vi "PKDAQInsertBlockData.vi"(0 "Block Data":T1, 5 "C12":dbl, 7 "C13L":dbl, 9 "C13H":dbl, 11 "Counts":u32, 12 "LT":dbl, 13 "RT":dbl) -> (4 "Block Data Out":T1)   [LabVIEW 2011]
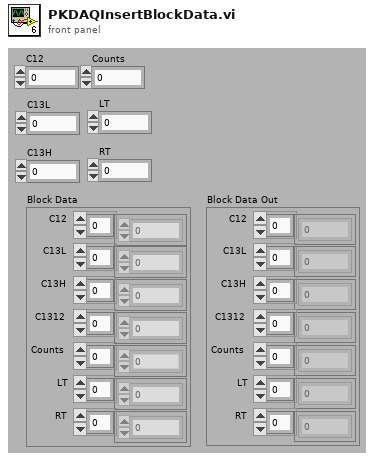
[diagram p1: front panel]
types:
  T1 = cluster{"C12":dbl[], "C13L":dbl[], "C13H":dbl[], "Counts":u32[], "LT":dbl[], "RT":dbl[], "C1312":dbl[]}
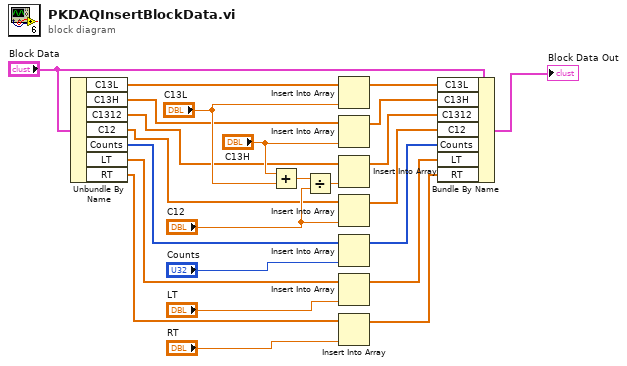
[diagram p0: block diagram]
diagram:
  n1 = Unbundle By Name("Block Data") -> ("C13L"=w4:dbl[], "C13H"=w1:dbl[], "C1312"=w3:dbl[], "C12"=w2:dbl[], "Counts"=w20:u32[], "LT"=w19:dbl[], "RT"=w18:dbl[])
  n2 = Add(x="C13H", y="C13L") -> (x+y=w10:dbl)
  n3 = Divide(x=w10, y="C12") -> (x/y=w9:dbl)
  n4 = Insert Into Array(array=w4, new element="C13L") -> (w5:dbl[])  [unwired: 1 in]
  n5 = Insert Into Array(array=w1, new element="C13H") -> (w6:dbl[])  [unwired: 1 in]
  n6 = Insert Into Array(array=w3, new element=w9) -> (w7:dbl[])  [unwired: 1 in]
  n7 = Insert Into Array(array=w2, new element="C12") -> (w8:dbl[])  [unwired: 1 in]
  n8 = Insert Into Array(array=w20, new element="Counts") -> (w17:u32[])  [unwired: 1 in]
  n9 = Insert Into Array(array=w19, new element="LT") -> (w16:dbl[])  [unwired: 1 in]
  n10 = Insert Into Array(array=w18, new element="RT") -> (w15:dbl[])  [unwired: 1 in]
  n11 = Bundle By Name(cluster="Block Data", "C13L"=w5, "C13H"=w6, "C1312"=w7, "C12"=w8, "Counts"=w17, "LT"=w16, "RT"=w15) -> (→"Block Data Out":T1)
